vi "New.vi"(8 "error in (no error)":errorcluster, 11 "UNSUBSCRIBE Request Data (JSON)":T1) -> (0 "error out":errorcluster, 3 "Unsubscribe JSON out":refnum<class "Unsubscribe JSON.lvclass">)   [LabVIEW 2020, in "wamplv.lvlib" / "Unsubscribe JSON.lvclass"]
uses:
  Unsubscribe JSON.lvclass
  WAMP Client/Private/TypeDef/UNSUBSCRIBE Request Data (JSON).ctl
  Unsubscribe JSON.lvclass/Unsubscribe JSON.ctl
  wamplv.lvlib
  Message loop classes/ErrorOrSuccess JSON/ErrorOrSuccess JSON.lvclass
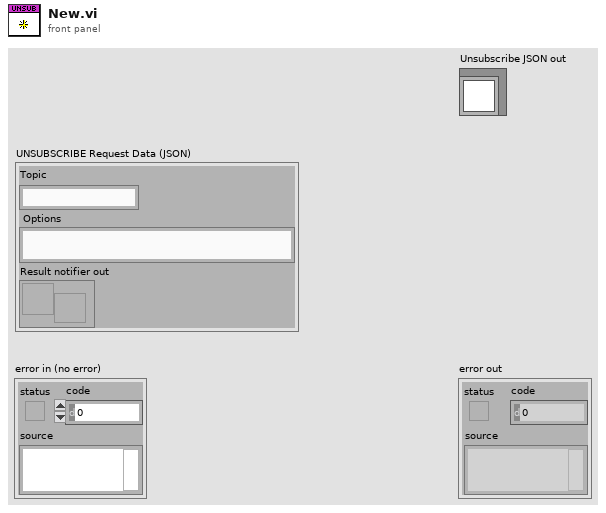
[diagram p1: front panel]
types:
  T1 = typedef "wamplv.lvlib/UNSUBSCRIBE Request Data (JSON).ctl" = cluster{"Topic":string, "Options":string, "Result notifier out":refnum<notifier>}
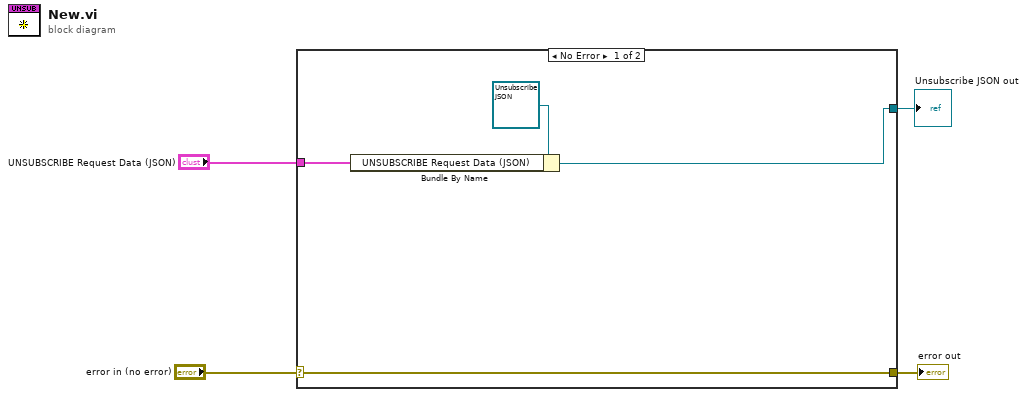
[diagram p0: block diagram]
diagram:
  n1 = case shown="No Error" "error in (no error)" {
    selector: "error in (no error)" -> [w8 w9]
    tunnel: [w8 w9] -> w3
    tunnel: [w6 _] -> w2
    tunnel: "UNSUBSCRIBE Request Data (JSON)" -> [w7 _]
    frame No Error {
      n2 = Bundle By Name(cluster=refnum<class "Unsubscribe JSON.lvclass"> refnum ("wamplv.lvlib:Unsubscribe JSON.lvclass"), "UNSUBSCRIBE Request Data (JSON)"=w7) -> (w6:refnum<class "Unsubscribe JSON.lvclass">)
    }
    frame Error {
    }
  }
  "error out" <- w3
  "Unsubscribe JSON out" <- w2
